vi "Build Application with API.vi"(8 "error in (no error)":errorcluster, 11 "PostBuildSupport in":refnum<class "PostBuildSupport.lvclass">) -> (0 "error out":errorcluster, 3 "PostBuildSupport out":refnum<class "PostBuildSupport.lvclass">)   [LabVIEW 2019, in "PostBuildSupport.lvclass"]
uses:
  PostBuildSupport.lvclass
  PostBuildSupport.lvclass/PostBuildSupport.ctl
  <vilib>/AppBuilder/AB_API/EXE/NI_AB_API_EXE.lvclass
panel:
  in  "Cancel Button":bool
  out "Progress Bar":u8(slide) caption="The build is complete. You can locate the build at\nC:\\user\\patrick\\git\\PPMS-Monitor-and-Control\\builds\\PPMS Monitor and Control\\Application." scale=0.0..100.0
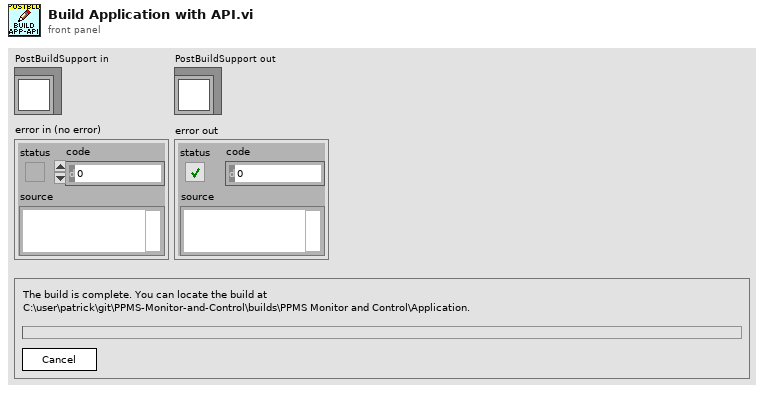
[diagram p1: front panel]
types:
  T1 = enum8{"Enabled", "Disabled", "Disabled and Grayed Out"}
  T2 = typedef "AB_API ProgressBar_Events.ctl" = cluster{"newJob":refnum<user-event>, "newItem":refnum<user-event>, "errorMsg":T3, "cancel":refnum<user-event>}
  T3 = typedef "AB_API ProgressBar_BuildError.ctl" = refnum<user-event>
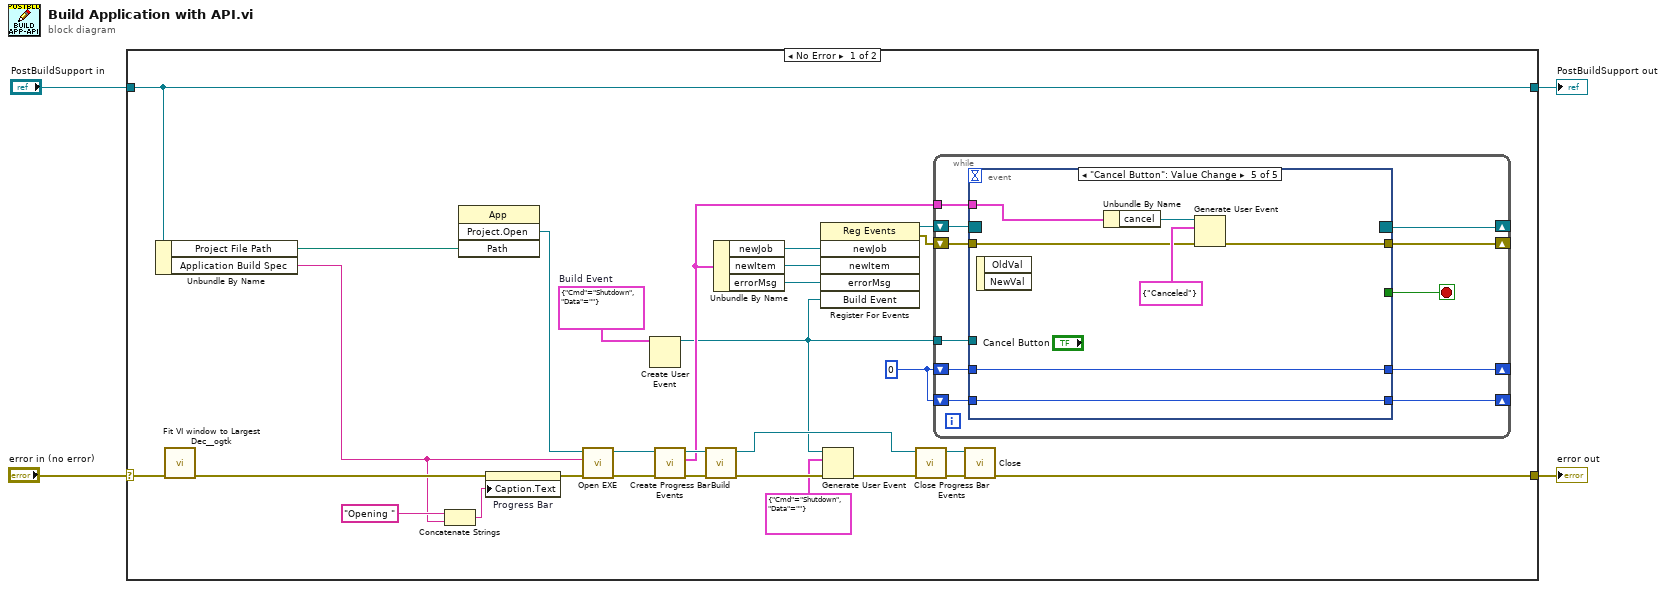
[diagram p0: block diagram]
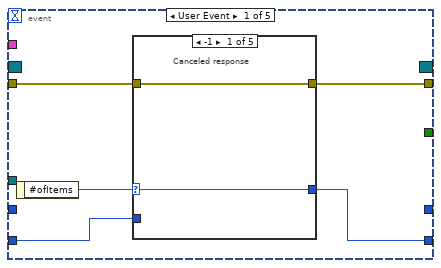
[diagram p2: hidden frame]
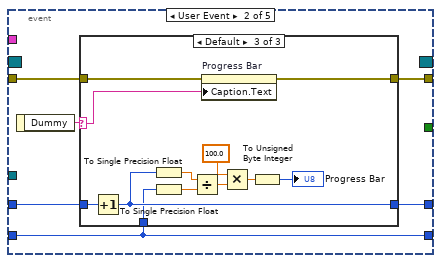
[diagram p7: hidden frame]
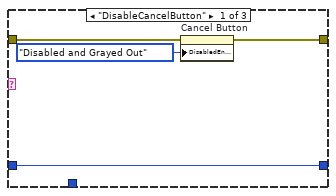
[diagram p8: hidden frame]
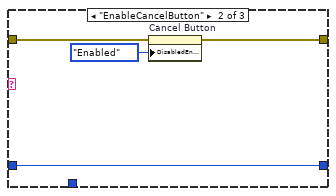
[diagram p9: hidden frame]
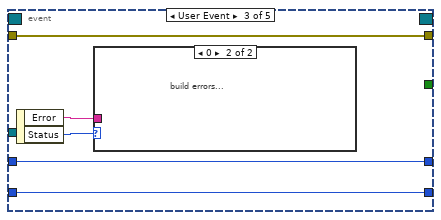
[diagram p10: hidden frame]
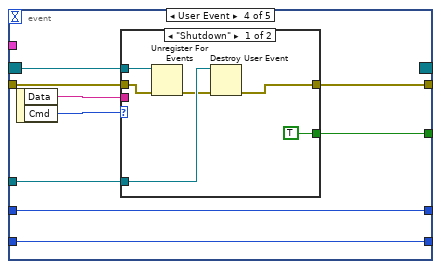
[diagram p12: hidden frame]
diagram:
  n1 = case shown="No Error" "error in (no error)" {
    selector: "error in (no error)" -> [w30 w115]
    tunnel: "PostBuildSupport in" -> [w33 w114]
    tunnel: [w32 w115] -> w2
    tunnel: [w33 w114] -> w1
    frame No Error {
      w19 = cluster{"Cmd":enum16{"Shutdown"}, "Data":string} {"Cmd"=enum."Shutdown", "Data"=""}  # Build Event
      w18 = 0 ("#ofItems")
      n2 = Unbundle By Name(w33) -> ("Project File Path"=w7:path, "Application Build Spec"=w5:string)
      n3 = call <userlib>:"Fit VI window to Largest Dec__ogtk.vi"("error in (no error)"=w30) -> ("error out"=w6:errorcluster)  [unwired: 5 in, 1 out]
      n4 = Concatenate Strings("Opening " ("string"), w5) -> (w9:string)
      n5 = invoke class="App" method="Project.Open"("Path"=w7) -> ("Project:Open"=w31:refnum<vi>)  [unwired: 3 in, 3 out]
      n6 = property on="Progress Bar" class="Slide (strict)"(error in=w6, "Caption.Text"=w9) -> (error out=w10:errorcluster)  [unwired: 1 in, 1 out]
      n7 = call <vilib>:"Open EXE.vi"("error in (no error)"=w10, "Build specification name"=w5, "Project Refnum"=w31) -> ("error out"=w11:errorcluster, "EXE out"=w12:refnum<class "NI_AB_API_EXE.lvclass">)  [unwired: 7 in]
      n8 = Create User Event(user event datatype=w19) -> (user event=w14:refnum<user-event>)  [unwired: 1 in, 1 out]
      n9 = call-dynamic "Create Progress Bar Events.vi"("error in (no error)"=w11, "NI_AB_API_Build in"=w12) -> ("error out"=w25:errorcluster, "progressBarEvents"=w17:T2, "NI_AB_API_Build out"=w29:refnum<class "NI_AB_API_EXE.lvclass">)  [unwired: 7 in]
      n10 = call-dynamic "Build.vi"("error in (no error)"=w25, "EXE in"=w29) -> ("error out"=w16:errorcluster, "EXE out"=w28:refnum<class "NI_AB_API_EXE.lvclass">)  [unwired: 6 in, 2 out]
      n11 = Unbundle By Name(w17) -> ("newJob"=w24:refnum<user-event>, "newItem"=w23:refnum<user-event>, "errorMsg"=w22:T3)
      n12 = register-events(w24, w23, w22, w14) -> (reference out=w21:refnum<event-registration>, error out=w20:errorcluster)  [unwired: 2 in]
      n13 = Generate User Event(user event=w14, event data cluster=cluster{"Cmd":enum16{"Shutdown"}, "Data":string} {"Cmd"=enum."Shutdown", "Data"=""} ("event data"), error in=w16) -> (error out=w15:errorcluster)  [unwired: 1 in, 1 out]
      n14 = call-dynamic "Close Progress Bar Events.vi"("error in (no error)"=w15, "NI_AB_API_Build in"=w28) -> ("error out"=w26:errorcluster, "NI_AB_API_Build out"=w27:refnum<class "NI_AB_API_EXE.lvclass">)  [unwired: 8 in]
      n15 = while {
        shift-right: [w44] -> _
        shift-left: w20 -> [w41]
        shift-right: [w43] -> _
        shift-left: w21 -> [w42]
        shift-right: [w39] -> _
        shift-left: w18 -> [w36]
        shift-right: [w38] -> _
        shift-left: w18 -> [w37]
        tunnel: w14 -> [w35]
        tunnel: w17 -> [w34]
        stop <- w40 stop-if-true
        n16 = event shown="[4] \"Cancel Button\": Value Change" {
          selector: w42 -> [_ _ _ w95 _]
          dyn-events: [_ _ _ _ _] -> w43
          timeout: _ -> [_ _ _ _ _]
          tunnel: [w48 w61 w90 w94 w111] -> w44
          tunnel: w41 -> [w49 w60 w90 w93 w107]
          tunnel: [_ _ _ w97 _] -> w40
          tunnel: [w46 w63 w88 w98 w110] -> w39
          tunnel: [_ w64 w89 w99 w109] -> w38
          tunnel: w37 -> [_ w62 w89 w99 w109]
          tunnel: w36 -> [w45 w63 w88 w98 w110]
          tunnel: w35 -> [_ _ _ w91 _]
          tunnel: w34 -> [_ _ _ _ w108]
          event User Event {
            n17 = event-data() -> ("#ofItems"=w47:i32)  [unwired: 1 in]
            n18 = case shown="-1" w47 {
              selector: w47 -> [w51 w53 w55 _ w59]
              tunnel: w49 -> [w50 w52 w54 w57 w58]
              tunnel: [w50 w52 w54 w57 w58] -> w48
              tunnel: [w51 w53 w55 w56 w59] -> w46
              tunnel: w45 -> [_ _ _ w56 _]
              frame -1 {
                # "Canceled response"
              }
              frame -2 {
              }
              frame -3 {
              }
              frame -4 {
              }
              frame Default {
              }
            }
          }
          event User Event {
            n19 = event-data() -> ("Dummy"=w65:string)  [unwired: 1 in]
            n20 = case shown="Default" w65 {
              selector: w65 -> [_ _ w76]
              tunnel: w62 -> [w68 w72 w83]
              tunnel: [w68 w72 w82] -> w64
              tunnel: w63 -> [_ _ w81]
              tunnel: [w66 w70 w74] -> w61
              tunnel: w60 -> [w67 w71 w75]
              frame "DisableCancelButton" {
                n21 = property on="Cancel Button" class="Bool"(error in=w67, "DisabledEnum"=T1."Disabled and Grayed Out" ("Disabled")) -> (error out=w66:errorcluster)  [unwired: 1 in, 1 out]
              }
              frame "EnableCancelButton" {
                n22 = property on="Cancel Button" class="Bool"(error in=w71, "DisabledEnum"=T1."Enabled" ("Disabled")) -> (error out=w70:errorcluster)  [unwired: 1 in, 1 out]
              }
              frame Default {
                n23 = Increment(x=w83) -> (x+1=w82:i32)
                n24 = To Single Precision Float(number=w82) -> (single precision float=w79:sgl)
                n25 = To Single Precision Float(number=w81) -> (single precision float=w78:sgl)
                n26 = Divide(x=w79, y=w78) -> (x/y=w80:sgl)
                n27 = property on="Progress Bar" class="Slide (strict)"(error in=w75, "Caption.Text"=w76) -> (error out=w74:errorcluster)  [unwired: 1 in, 1 out]
                n28 = Multiply(x=sgl 100.0, y=w80) -> (x*y=w85:sgl)
                n29 = To Unsigned Byte Integer(number=w85) -> (unsigned 8bit integer=→"Progress Bar":u8)
              }
            }
          }
          event User Event {
            n30 = event-data() -> ("Error"=w86:string, "Status"=w87:i32)  [unwired: 1 in]
            n31 = case shown="0" w87 {
              tunnel: w86 -> [_ _]
              frame Default {
              }
              frame 0 {
                # "build errors..."
              }
            }
          }
          event User Event {
            n32 = event-data() -> ("Data"=w92:string, "Cmd"=w96:enum16{"Shutdown"})  [unwired: 1 in]
            n33 = case shown="\"Shutdown\"" w96 {
              tunnel: [TRUE _] -> w97
              tunnel: w95 -> [w104 _]
              tunnel: [w100 w106] -> w94
              tunnel: w93 -> [w103 w106]
              tunnel: w92 -> [_ _]
              tunnel: w91 -> [w102 _]
              frame "Shutdown" {
                n34 = Unregister For Events(event registration refnum=w104, error in=w103) -> (error out=w101:errorcluster)
                n35 = Destroy User Event(user event=w102, error in=w101) -> (error out=w100:errorcluster)
              }
              frame Default {
              }
            }
          }
          event "Cancel Button": Value Change {
            n36 = event-data() -> ()  [unwired: 1 in, 2 out]
            n37 = Unbundle By Name(w108) -> ("cancel"=w112:refnum<user-event>)
            n38 = Generate User Event(user event=w112, event data cluster=cluster{"Dummy":string} {"Dummy"="Canceled"} ("event data"), error in=w107) -> (error out=w111:errorcluster)  [unwired: 1 in, 1 out]
          }
        }
      }
      n39 = call-dynamic "Close.vi"("error in (no error)"=w26, "EXE in"=w27) -> ("error out"=w32:errorcluster)  [unwired: 9 in]
    }
    frame Error {
    }
  }
  "error out" <- w2
  "PostBuildSupport out" <- w1
